vi "Read active scale index .vi"(8 "error in (no error)":errorcluster, 11 "Scaling editor node in":refnum<class "Scaling editor node.lvclass">) -> (0 "error out":errorcluster, 2 "active scale index":i32, 3 "Scaling editor node out":refnum<class "Scaling editor node.lvclass">)   [LabVIEW 2013, in "Scaling editor node.lvclass"]
uses:
  Scaling editor node.lvclass
  Scaling editor node.lvclass/Scaling editor node.ctl
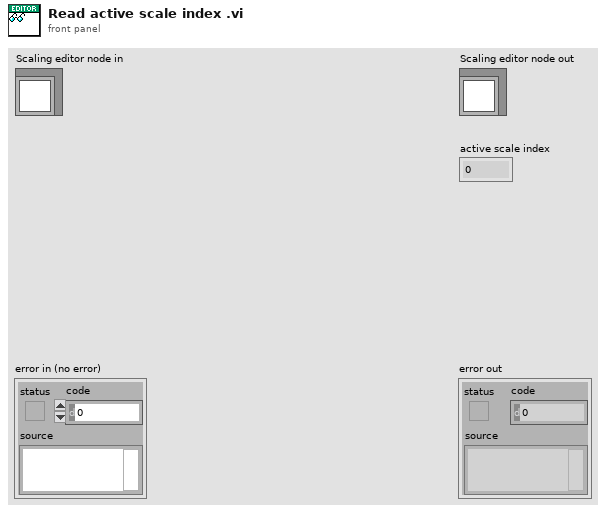
[diagram p1: front panel]
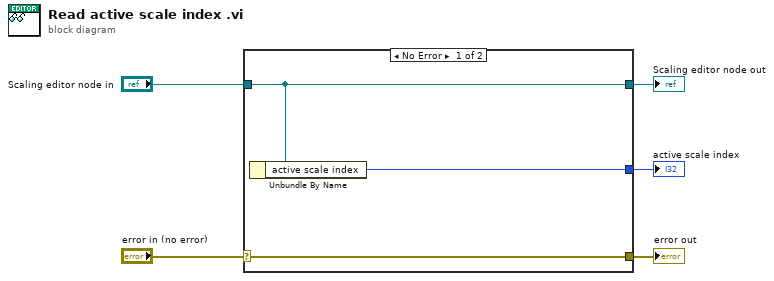
[diagram p0: block diagram]
diagram:
  n1 = case shown="No Error" "error in (no error)" {
    selector: "error in (no error)" -> [w8 w9]
    tunnel: [w8 w9] -> w4
    tunnel: [w7 w10] -> w2
    tunnel: "Scaling editor node in" -> [w7 w10]
    tunnel: [w6 _] -> w1
    frame No Error {
      n2 = Unbundle By Name(w7) -> ("active scale index"=w6:i32)
    }
    frame Error {
    }
  }
  "error out" <- w4
  "Scaling editor node out" <- w2
  "active scale index" <- w1
